vi "LNAttenuation Group.vi"(3 "Upper Threshold (% of Max)":dbl=80.0, 6 "data":dbl[][](array[numeric]), 7 "Lower Threshold (% of Min)":dbl=120.0) -> (12 "LN Attenuation1":dbl, 13 "LN Attenuation 2":dbl, 14 "Upper Voltage Threshold Channel 1":dbl, 15 "Lower Voltage Threshold Channel 1":dbl, 16 "Upper Voltage Threshold Reference":dbl, 17 "Lower Voltage Threshold Reference":dbl, 18 "Upper Voltage Threshold Signal 2":dbl, 19 "Lower Voltage Threshold Signal 2":dbl)   [LabVIEW 2009]
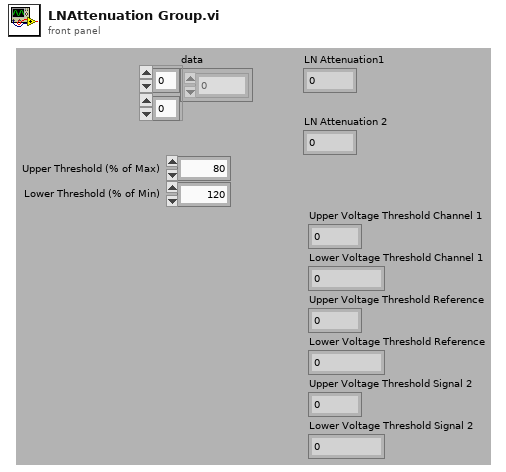
[diagram p1: front panel]
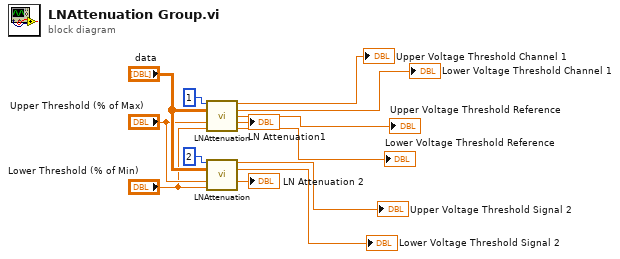
[diagram p0: block diagram]
diagram:
  n1 = call "LNAttenuation.vi"("index (row)"=1, "data"="data", "Upper Threshold (% of Max)"="Upper Threshold (% of Max)", "Lower Threshold (% of Min)"="Lower Threshold (% of Min)") -> ("Upper Voltage Threshold Signal"=→"Upper Voltage Threshold Channel 1":dbl, "Lower Voltage Threshold Signal"=→"Lower Voltage Threshold Channel 1":dbl, "Upper Voltage Threshold Ref"=→"Upper Voltage Threshold Reference":dbl, "LN Attenuation"=→"LN Attenuation1":dbl, "Lower Voltage Threshold Ref"=→"Lower Voltage Threshold Reference":dbl)  [unwired: 7 in]
  n2 = call "LNAttenuation.vi"("index (row)"=2, "data"="data", "Upper Threshold (% of Max)"="Upper Threshold (% of Max)", "Lower Threshold (% of Min)"="Lower Threshold (% of Min)") -> ("Upper Voltage Threshold Signal"=→"Upper Voltage Threshold Signal 2":dbl, "Lower Voltage Threshold Signal"=→"Lower Voltage Threshold Signal 2":dbl, "LN Attenuation"=→"LN Attenuation 2":dbl)  [unwired: 7 in, 2 out]
